vi "Invalid Priority.vi"(7 "error source vi name":string, 8 "error in (no error)":errorcluster, 10 "priority":u64, 11 "Timing in":refnum<class "Timing.lvclass">) -> (0 "error out":errorcluster, 3 "Timing out":refnum<class "Timing.lvclass">)   [LabVIEW 2019, in "DSF Core.lvlib" / "Timing.lvclass"]
uses:
  Timing.lvclass
  Errors.ctl
  <vilib>/NI/Memory Manager/VIs/Write Numeric Scalar to Source (Base10 U64).vi
  <vilib>/NI/Memory Manager/VIs/New Error Cluster.vi
  <vilib>/NI/Memory Manager/VIs/New Error Cluster (512B).vi
  <vilib>/NI/Memory Manager/VIs/Set Error Code.vi
  <vilib>/NI/Memory Manager/VIs/Set Error Status.vi
  <vilib>/NI/Memory Manager/VIs/Set Error Source.vi
  VIs/Constants/Constants.vi
  VIs/Constants/Engine Library Name.vi
  Timing Error Info.vi
  VIs/Constants/Base Error Code.vi
  Base Error Offset.vi
  <vilib>/NI/Memory Manager/Static Errors.lvlib
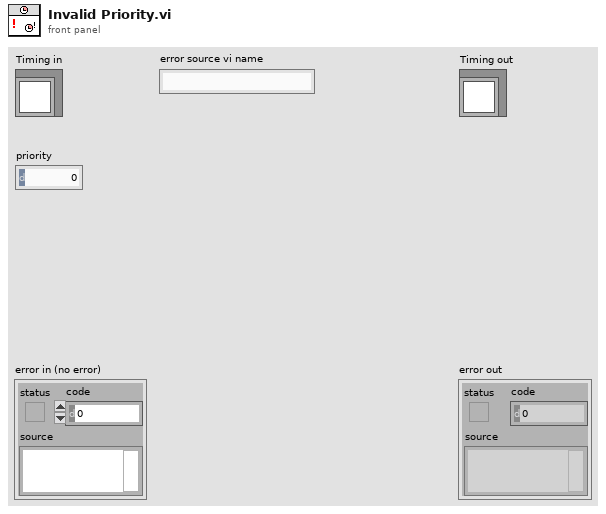
[diagram p1: front panel]
types:
  T1 = typedef "DSF Core.lvlib/Timing.lvclass/Errors.ctl" = enum16{"Invalid Offset", "Invalid Priority"}
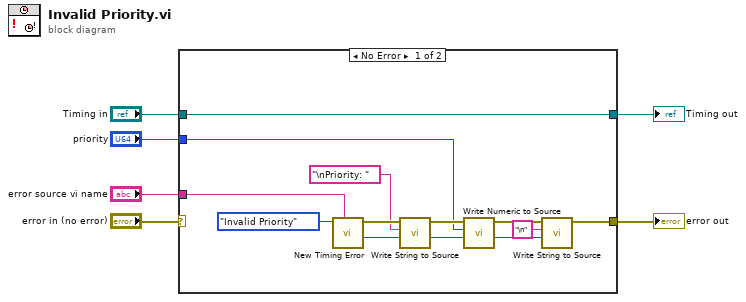
[diagram p0: block diagram]
diagram:
  n1 = case shown="No Error" "error in (no error)" {
    selector: "error in (no error)" -> [_ w20]
    tunnel: "Timing in" -> [w17 w21]
    tunnel: [w17 w21] -> w4
    tunnel: [w14 w20] -> w3
    tunnel: "error source vi name" -> [w18 _]
    tunnel: "priority" -> [w7 _]
    frame No Error {
      n2 = call "New Timing Error.vi"("error source vi name"=w18, "error"=Errors."Invalid Priority") -> ("new offset"=w13:i32, "error out"=w16:errorcluster)  [unwired: 8 in]
      n3 = call <vilib>:"Write String to Source.vi"("offset"=w13, "string"="\nPriority: ", "error in"=w16) -> ("new offset"=w12:i32, "error out"=w15:errorcluster)  [unwired: 7 in]
      n4 = call-poly <vilib>:"Write Numeric to Source.vi"("offset"=w12, "value"=w7, "error in"=w15) -> ("new offset"=w11:i32, "error out"=w8:errorcluster)  [unwired: 7 in]
      n5 = call <vilib>:"Write String to Source.vi"("offset"=w11, "string"="\n", "error in"=w8) -> ("error out"=w14:errorcluster)  [unwired: 7 in, 1 out]
    }
    frame Error {
    }
  }
  "error out" <- w3
  "Timing out" <- w4
